vi "Recursive Folder List2.vi"(4 "Folders to Exclude\nREP ( ^[_.] as Default)\nempty to disable this feature":string="^[_.]", 6 "pattern":string, 8 "error in (no error)":errorcluster, 9 "Continue Recursing on Error? (F)":bool, 11 "Folder Path":path) -> (0 "error out":errorcluster, 1 "Number of Folders":i32, 2 "All Folders":path[](array[path]), 3 "dup Folder Path":path)   [LabVIEW 2017]
doc: "Lists the contents of a folder or LLB."
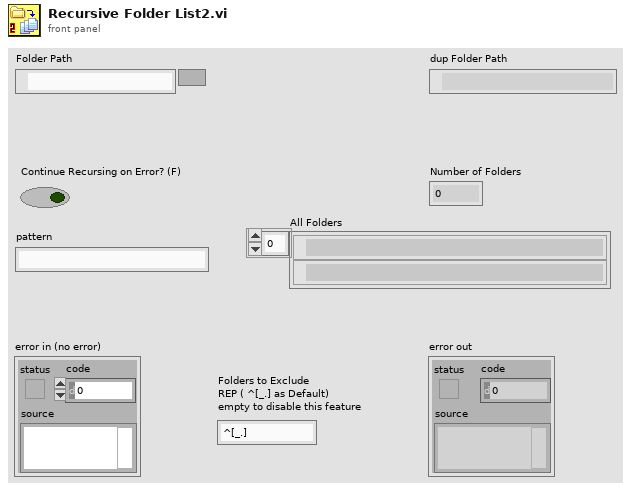
[diagram p1: front panel]
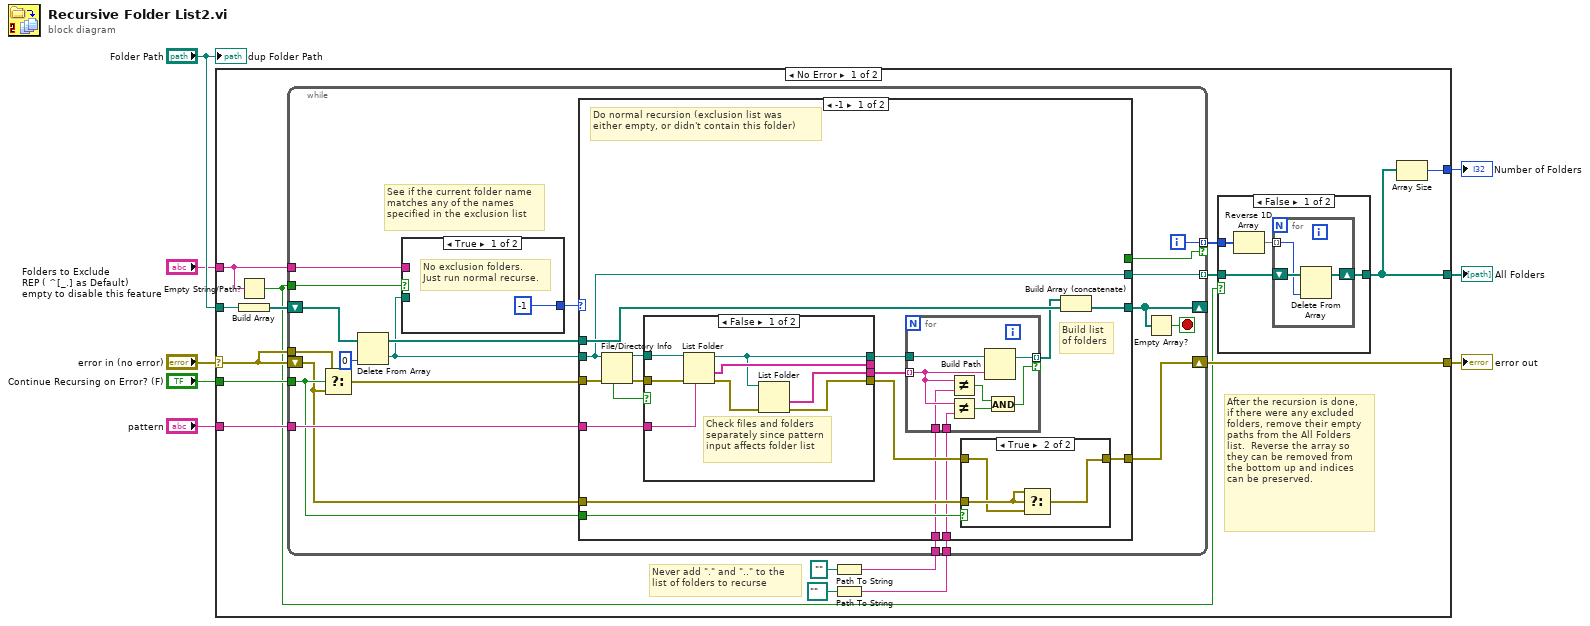
[diagram p0: block diagram]
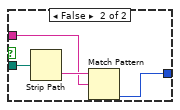
[diagram p2: hidden frame]
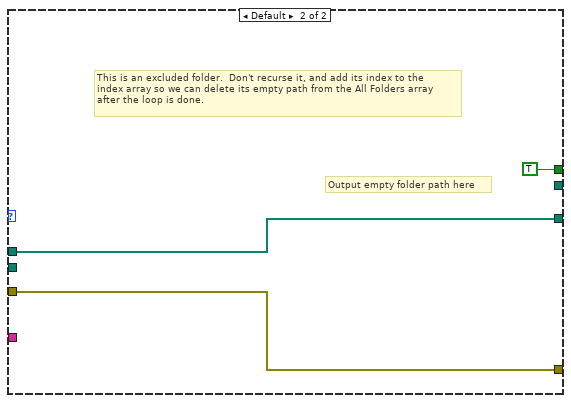
[diagram p5: hidden frame]
diagram:
  n1 = case shown="No Error" "error in (no error)" {
    selector: "error in (no error)" -> [w18 w100]
    tunnel: "Folder Path" -> [w24 _]
    tunnel: [w20 _] -> w8
    tunnel: [w21 w100] -> w7
    tunnel: [w9 _] -> w5
    tunnel: "pattern" -> [w22 _]
    tunnel: "Continue Recursing on Error? (F)" -> [w19 _]
    tunnel: "Folders to Exclude\nREP ( ^[_.] as Default)\nempty to disable this feature" -> [w10 _]
    frame No Error {
      # "Never add \".\" and \"..\" to the list of folders to recurse"
      # "After the recursion is done,\nif there were any excluded\nfolders, remove their empty\npaths from the All Folders\nlist.  Reverse the array so\nthey can be removed from\nthe bottom up and indices\ncan be preserved."
      n2 = Empty String/Path?(string/path=w10) -> (empty?=w11:bool)
      n3 = Build Array(w24) -> (w23:path[])
      n4 = Path To String(path=path "") -> (string=w13:string)
      n5 = Path To String(path=path "..") -> (string=w12:string)
      n6 = while {
        shift-left: w23 -> [w44]
        shift-right: [w42] -> _
        shift-right: [w36] -> w21
        shift-left: w18 -> [w35]
        tunnel: [w33] -> w17 mode=indexing
        tunnel: w22 -> [w43]
        tunnel: w19 -> [w37]
        tunnel: w18 -> [w38]
        tunnel: w10 -> [w31]
        tunnel: w11 -> [w32]
        tunnel: [w28] -> w16 mode=indexing if=w27
        tunnel: w13 -> [w26]
        tunnel: w12 -> [w25]
        i -> [w28]
        stop <- w41 stop-if-true
        # "See if the current folder name\nmatches any of the names\nspecified in the exclusion list"
        n7 = Select(t=w38, s=w37, f=w35) -> (s? t:f=w39:errorcluster)
        n8 = Delete From Array(array=w44, index=0) -> (deleted portion=w30:path, array with subset deleted=w34:path[])  [unwired: 1 in]
        n9 = case shown="True" w32 {
          tunnel: w31 -> [_ w47]
          tunnel: w30 -> [_ w49]
          tunnel: [-1 ("index of element") w46] -> w29
          frame True {
            # "No exclusion folders.\nJust run normal recurse."
          }
          frame False {
            n10 = Strip Path(path=w49) -> (name=w48:string)  [unwired: 1 out]
            n11 = Match Pattern(string=w48, regular expression=w47) -> (offset past match=w46:i32)  [unwired: 1 in, 3 out]
          }
        }
        n12 = case shown="-1" w29 {
          tunnel: w43 -> [w65 _]
          tunnel: [w63 w91] -> w42
          tunnel: w30 -> [w53 _]
          tunnel: w39 -> [w59 w90]
          tunnel: w37 -> [w57 _]
          tunnel: [w56 w90] -> w36
          tunnel: w35 -> [w55 _]
          tunnel: w34 -> [w54 w91]
          tunnel: [w53 _] -> w33
          tunnel: [_ TRUE] -> w27
          tunnel: w26 -> [w51 _]
          tunnel: w25 -> [w50 _]
          frame -1 {
            # "Build list\nof folders"
            # "Do normal recursion (exclusion list was\neither empty, or didn't contain this folder)"
            n13 = File/Directory Info(path=w53, error in=w59) -> (path out=w61:path, error out=w62:errorcluster, shortcut=w60:bool)  [unwired: 4 out]
            n14 = case shown="False" w60 {
              tunnel: [w82 _] -> _
              tunnel: [w81 w84] -> w66
              tunnel: [w80 w83] -> w58
              tunnel: w65 -> [w79 _]
              tunnel: [w75 _] -> w64
              tunnel: w62 -> [w78 w83]
              tunnel: w61 -> [w77 w84]
              frame False {
                # "Check files and folders\nseparately since pattern\ninput affects folder list"
                n15 = List Folder(path=w77, pattern=w79, error in=w78) -> (path out=w81:path, folder names=w82:string[], error out=w76:errorcluster)  [unwired: 2 out]
                n16 = List Folder(path=w81, error in=w76) -> (folder names=w75:string[], error out=w80:errorcluster)  [unwired: 4 out]
              }
              frame True {
                # "Do not attempt to recurse the contents of folder shortcuts"
              }
            }
            n17 = for {
              tunnel: w66 -> [w74]
              tunnel: [w73] -> w52 mode=indexing if=w72
              tunnel: w64 -> [w71] mode=indexing
              tunnel: w51 -> [w70]
              tunnel: w50 -> [w69]
              n18 = Not Equal?(x=w71, y=w70) -> (x != y?=w67:bool)
              n19 = Not Equal?(x=w71, y=w69) -> (x != y?=w68:bool)
              n20 = Build Path(base path=w74, name or relative path=w71) -> (appended path=w73:path)
              n21 = And(x=w67, y=w68) -> (x .and. y?=w72:bool)
            }
            n22 = case shown="True" w57 {
              tunnel: w58 -> [w85 w87]
              tunnel: [w85 w86] -> w56
              tunnel: w55 -> [_ w88]
              frame False {
              }
              frame True {
                n23 = Select(t=w88, s=w88, f=w87) -> (s? t:f=w86:errorcluster)
              }
            }
            n24 = Build Array (concatenate)(w52, w54) -> (w63:path[])
          }
          frame Default {
            # "Output empty folder path here"
            # "This is an excluded folder.  Don't recurse it, and add its index to the\nindex array so we can delete its empty path from the All Folders array\nafter the loop is done."
          }
        }
        n25 = Empty Array?(array=w42) -> (empty?=w41:bool)
      }
      n26 = case shown="False" w11 {
        tunnel: w17 -> [w94 w99]
        tunnel: [w93 w99] -> w9
        tunnel: w16 -> [w95 _]
        frame False {
          n27 = Reverse 1D Array(array=w95) -> (reversed array=w92:i32[])
          n28 = for {
            shift-right: [w97] -> w93
            shift-left: w94 -> [w98]
            tunnel: w92 -> [w96] mode=indexing
            n29 = Delete From Array(array=w98, index=w96) -> (array with subset deleted=w97:path[])  [unwired: 1 in, 1 out]
          }
        }
        frame True {
          # "No excluded folders.\nDon't run the code that\ndeletes excluded folder\nindices."
        }
      }
      n30 = Array Size(array=w9) -> (size(s)=w20:i32)
    }
    frame Error {
    }
  }
  "Number of Folders" <- w8
  "error out" <- w7
  "All Folders" <- w5
  "dup Folder Path" <- "Folder Path"
